vi "LV SciSDK DIGITIZER STOP.vi"(8 "error in (no error)":errorcluster, 9 "Digitizer Handle In":T1) -> (0 "error out":errorcluster, 1 "Digitizer Handle Out":T1)   [LabVIEW 2021]
uses:
  SciSDK_Labview.lvlib
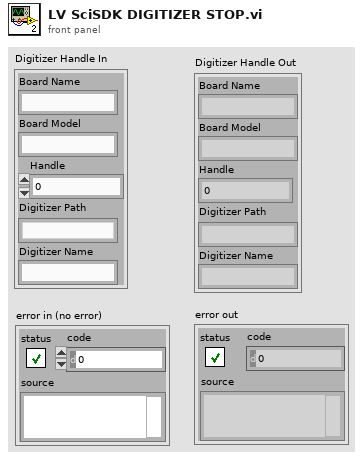
[diagram p1: front panel]
types:
  T1 = cluster{"Board Name":string, "Board Model":string, "Handle":u64, "Digitizer Path":string, "Digitizer Name":string}
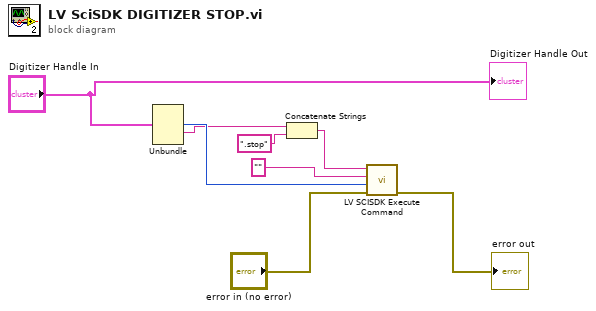
[diagram p0: block diagram]
diagram:
  n1 = Unbundle("Digitizer Handle In") -> ("Handle"=w7:u64, "Digitizer Path"=w6:string)  [unwired: 3 out]
  n2 = Concatenate Strings(w6, ".stop" ("string")) -> (w4:string)
  n3 = call "LV SCISDK Execute Command.vi"("error in (no error)"="error in (no error)", "handle"=w7, "value"="", "Path"=w4) -> ("error out"=→"error out":errorcluster)  [unwired: 5 in, 2 out]
  "Digitizer Handle Out" <- "Digitizer Handle In"
